vi "JoystickButtons.vi"(0 "Buttons":bool[](array[boolean])) -> (16 "10":bool, 17 "12":bool, 18 "9":bool, 19 "11":bool, 20 "1":bool, 21 "2":bool, 22 "3":bool, 23 "4":bool, 24 "5":bool, 25 "6":bool, 26 "7":bool, 27 "8":bool)   [LabVIEW 2015]
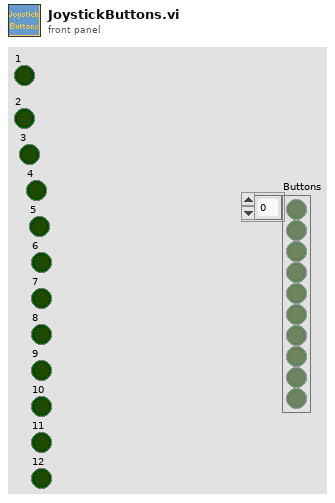
[diagram p1: front panel]
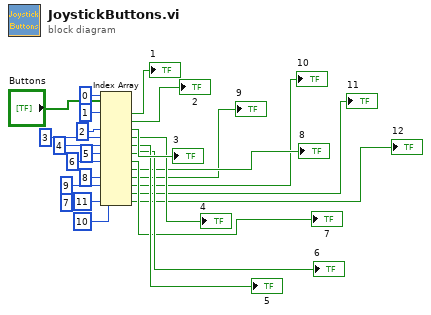
[diagram p0: block diagram]
diagram:
  n1 = Index Array(array="Buttons", index #1=0 ("index"), index #2=1 ("index"), index #3=2 ("index"), index #4=3 ("index"), index #5=4 ("index"), index #6=5 ("index"), index #7=6 ("index"), index #8=7 ("index"), index #9=8 ("index"), index #10=9 ("index"), index #11=10 ("index"), index #12=11 ("index")) -> (element #1=→"1":bool, element #2=→"2":bool, element #3=→"3":bool, element #4=→"4":bool, element #5=→"5":bool, element #6=→"6":bool, element #7=→"7":bool, element #8=→"8":bool, element #9=→"9":bool, element #10=→"10":bool, element #11=→"11":bool, element #12=→"12":bool)
